vi "Reference Origin.vi"(8 "error in (no error)":errorcluster, 9 "Pane":refnum<vi>, 10 "This VI":refnum<vi>, 11 "This Application":refnum<vi>) -> (0 "error out":errorcluster, 3 "DAQ Type":enum16{"Hardware", "Simulation"}(ring))   [LabVIEW 2021, in "User Interface.lvlib"]
uses:
  User Interface.lvlib
  <vilib>/Utility/miscctls.llb/LVPointTypeDef.ctl
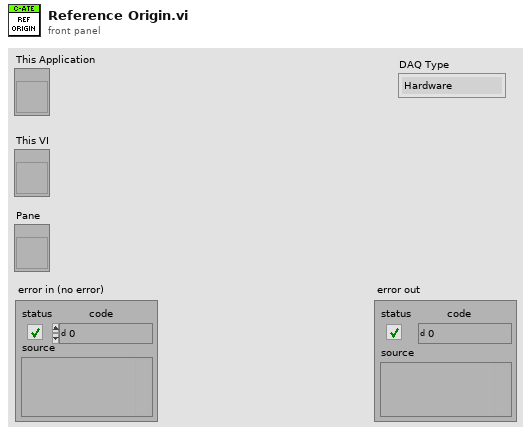
[diagram p1: front panel]
types:
  T1 = enum32{"invalid app kind", "Development System", "Run Time System", "Student Edition", "Embedded LabVIEW", "Evaluation", "Custom"}
  T2 = typedef "LVPointTypeDef.ctl" = cluster{"Horizontal":i16, "Vertical":i16}
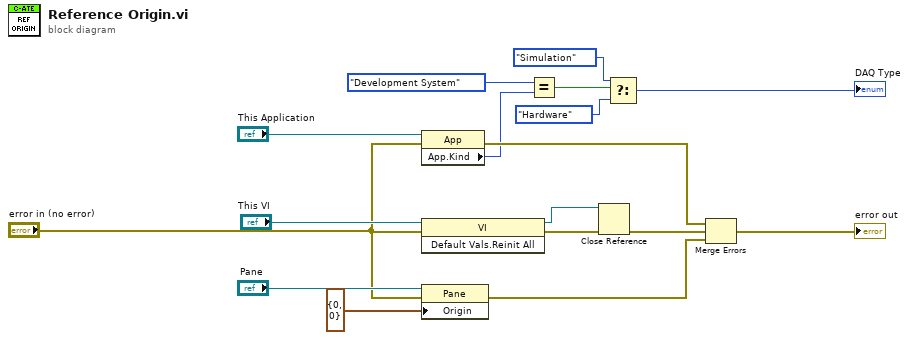
[diagram p0: block diagram]
diagram:
  n1 = property class="App"(reference="This Application", error in="error in (no error)") -> (error out=w8:errorcluster, "App.Kind"=w7:T1)  [unwired: 1 out]
  n2 = invoke class="VI" method="Default Vals.Reinit All"(reference="This VI", error in="error in (no error)") -> (reference out=w15:refnum<vi>, error out=w16:errorcluster)  [unwired: 1 in, 1 out]
  n3 = property class="Pane"(reference="Pane", error in="error in (no error)", "Origin"=T2 {"Horizontal"=0, "Vertical"=0}) -> (error out=w12:errorcluster)  [unwired: 1 out]
  n4 = Equal?(x=T1."Development System" ("Application:Kind"), y=w7) -> (x = y?=w5:bool)
  n5 = Close Reference(reference=w15, error in (no error)=w16) -> (error out=w9:errorcluster)
  n6 = Select(t=enum16{"Hardware", "Simulation"}."Simulation" ("DAQ Type"), s=w5, f=enum16{"Hardware", "Simulation"}."Hardware" ("DAQ Type")) -> (s? t:f=→"DAQ Type":enum16{"Hardware", "Simulation"})
  n7 = Merge Errors(w8, w9, w12) -> (→"error out":errorcluster)
